vi "JSON to LVObject - Aggregate Descendant And JSON Object With All Fields - Returns Aggregate Descendant With All Fields Set.vi"() -> ()   [LabVIEW 2017, in "Tests.lvlib"]
uses:
  Tests.lvlib
  Flatten To JSON Object/Flatten To JSON Object.lvclass
  City/City.lvclass
  Temperature Forecast/Temperature Forecast.lvclass
  C:/Users/de200256/Code/logmanoriginal/jsontext-object-serialization/Tests/Weather Forecast/Weather Forecast.lvclass
  <vilib>/addons/_JKI Toolkits/Caraya/classes/Assert/Assert Equal Value and Type_Variant.vi
  <vilib>/addons/_JKI Toolkits/Caraya/classes/Test/Test.lvclass
  <vilib>/addons/_JKI Toolkits/Caraya/classes/Assert/Assert.lvclass
panel:
  out "error out":errorcluster
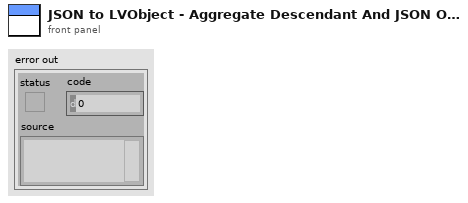
[diagram p1: front panel]
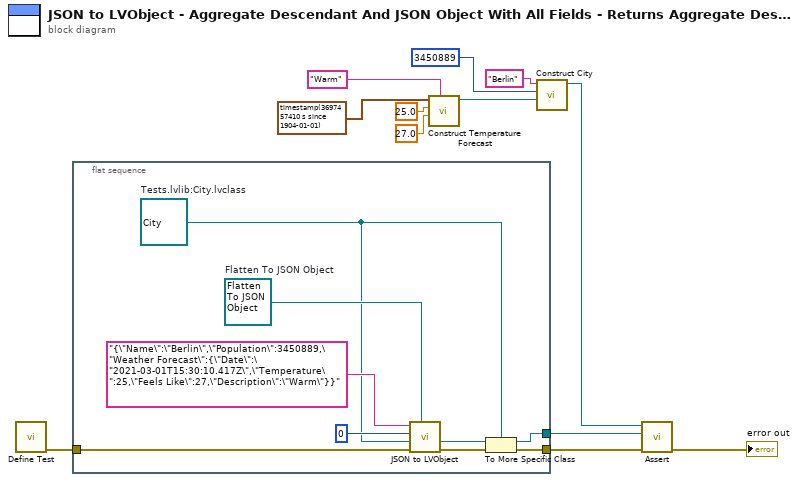
[diagram p0: block diagram]
diagram:
  n1 = call <vilib>:"Define Test.vi"() -> ("error out"=w12:errorcluster)  [unwired: 11 in]
  n2 = flat-sequence {
    tunnel: w12 -> [w20]
    tunnel: [w16] -> w11
    tunnel: [w13] -> w10
    frame #0 {
      w14 = refnum<class "City.lvclass"> refnum  # Tests.lvlib:City.lvclass
      w21 = refnum<class "Flatten To JSON Object.lvclass"> refnum  # Flatten To JSON Object
      n3 = call-dynamic "JSON to LVObject.vi"("Flatten To JSON Object in"=w21, "error in (no error)"=w20, "Object Type"=w14, "Offset"=0, "JSON"="{\"Name\":\"Berlin\",\"Population\":3450889,\"Weather Forecast\":{\"Date\":\"2021-03-01T15:30:10.417Z\",\"Temperature\":25,\"Feels Like\":27,\"Description\":\"Warm\"}}") -> ("error out"=w19:errorcluster, "Object"=w15:refnum<class>)  [unwired: 5 in]
      n4 = To More Specific Class(target class=w14, reference=w15, error in=w19) -> (specific class reference=w13:refnum<class "City.lvclass">, error out=w16:errorcluster)
    }
  }
  n5 = call "Construct Temperature Forecast.vi"("Description"="Warm", "Feels Like [°C]"=27.0, "Temperature [°C]"=25.0, "Date"=timestamp(3697457410.417 s since 1904-01-01)) -> ("Temperature Forecast"=w2:refnum<class "Temperature Forecast.lvclass">)  [unwired: 6 in, 1 out]
  n6 = call "Construct City.vi"("Weather Forecast"=w2, "Population"=u32 3450889, "Name"="Berlin") -> ("City"=w1:refnum<class "City.lvclass">)  [unwired: 7 in, 1 out]
  n7 = call-poly <vilib>:"Assert.vi"("error in (no error)"=w11, "Y"=w10, "X"=w1) -> ("error out"=→"error out":errorcluster)  [unwired: 8 in]
